vi "AutoHelperDelayedAction_Example.vi"() -> ()   [LabVIEW 2019]
uses:
  <vilib>/Rock Robotics/WPI/ThirdParty/JAS_Junk/TrajLib/VI/Util_GetTime_U32.vi
  <vilib>/Rock Robotics/WPI/ThirdParty/JAS_Junk/TrajLib/VI/DigSeqLogic_Edge_On.vi
  <vilib>/Rock Robotics/WPI/ThirdParty/JAS_Junk/TrajLib/Timer_New.vi
  <vilib>/Rock Robotics/WPI/ThirdParty/JAS_Junk/TrajLib/DigSeqLogic_SR_FlipFlop.vi
  <vilib>/Rock Robotics/WPI/ThirdParty/JAS_Junk/TrajLib/DigSeqLogic_Off_Delay.vi
  <vilib>/Rock Robotics/WPI/ThirdParty/JAS_Junk/TrajLib/VI/Util_GetTime_U64.vi
  <vilib>/Utility/semaphor.llb/Obtain Semaphore Reference.vi
  <vilib>/Rock Robotics/WPI/ThirdParty/JAS_Junk/TrajLib/Timer_Reset.vi
  <vilib>/Rock Robotics/WPI/ThirdParty/JAS_Junk/TrajLib/Timer_Start.vi
  <vilib>/Rock Robotics/WPI/ThirdParty/JAS_Junk/TrajLib/Timer_HasPeriodPassedOnce.vi
  <vilib>/Rock Robotics/WPI/ThirdParty/JAS_Junk/TrajLib/Timer_Stop.vi
  <vilib>/Rock Robotics/WPI/ThirdParty/JAS_Junk/TrajLib/VI/Timer_Restart.vi
  <vilib>/Rock Robotics/WPI/ThirdParty/JAS_Junk/TrajLib/Trajectory_Library.lvlib
panel:
  out "Remaining\nTime":dbl format="%12.2f"
  in  "Step Start":bool
  out "Waveform Chart":cluster{i16, i16}(graph)
  out "Delayed Action":bool
  out "Step Start FB":bool
  in  "Delay (sec)":dbl=600.0
  # "AUTO HELPER DELAYED ACTION"
  # "THIS LIBRARY VI IS A WORK IN PROGRESS"
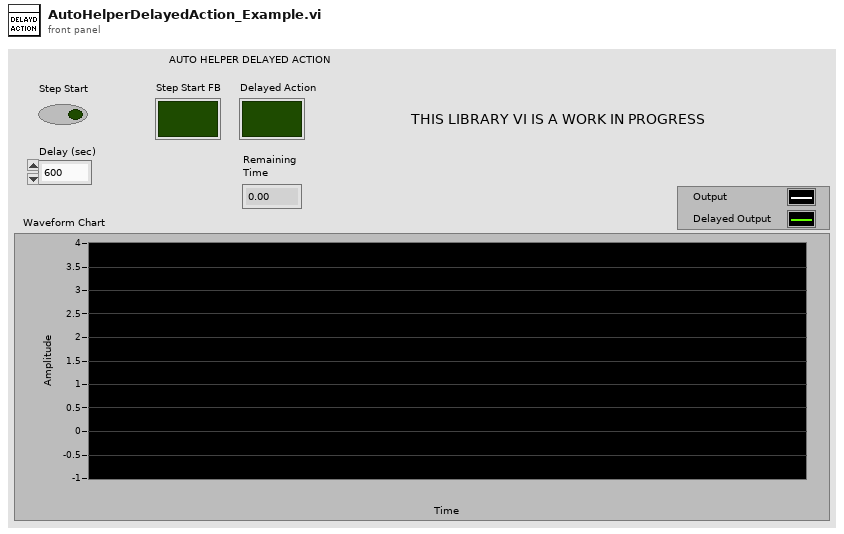
[diagram p1: front panel]
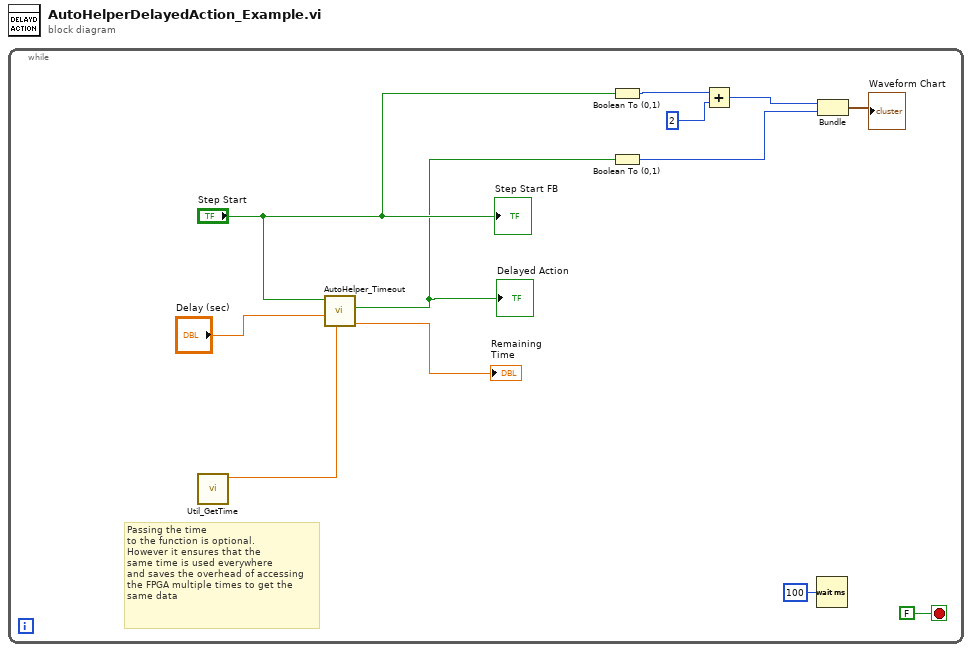
[diagram p0: block diagram]
diagram:
  n1 = while {
    stop <- FALSE stop-if-true
    # "Passing the time\nto the function is optional.\nHowever it ensures that the\nsame time is used everywhere\nand saves the overhead of accessing\nthe FPGA multiple times to get the\nsame data"
    n2 = call <vilib>:"Util_GetTime.vi"() -> ("FPGA_Time_Seconds"=w4:dbl)  [unwired: 9 in, 2 out]
    n3 = call <vilib>:"AutoHelper_Timeout.vi"("Pass_Through_Time"=w4, "Timeout Sec"="Delay (sec)", "New Step"="Step Start") -> ("Remaining ALT"=→"Remaining\nTime":dbl, "Timeout ALT"=w2:bool)  [unwired: 5 in, 2 out]
    "Delayed Action" <- w2
    n4 = Boolean To (0,1)(Boolean="Step Start") -> (0, 1=w8:i16)
    n5 = Boolean To (0,1)(Boolean=w2) -> (0, 1=w6:i16)
    n6 = Add(x=w8, y=i16 2) -> (x+y=w7:i16)
    n7 = Wait (ms)(milliseconds to wait=u32 100) -> ()  [unwired: 1 out]
    n8 = Bundle(w7, w6) -> (→"Waveform Chart":cluster{i16, i16})  [unwired: 1 in]
    "Step Start FB" <- "Step Start"
  }
